vi "AutoReadFile.vi"(8 "error in (no error)":errorcluster, 11 "FileName":string="trajectory.csv") -> (0 "error out":errorcluster, 3 "outTRAJECTORY":T1[](array[typedef]), 4 "Full FIlename":string)   [LabVIEW 2023]
doc: "Create a trajectory from a CSV file. This can be used on a PC or the RoboRIO. Normally the CSV file is created as output from one of the trajectory utility programs. The file could also be created manually or by a custom written program.\n\nParameters:\n - FileName -- Name of the CSV file to read. See file name notes for additional information.\n - Error In -- Input error cluster (optional)\n\nReturns:\n - outTrajectory - Trajectory data structure cluster\n - Error out - returned error cluster\n\nNotes on use:\n -- This routine writes informational messges to the console and to the driver station log.\n\nNotes on file naming:\n -- The file name must include the extention. \".csv\" is not automatically appended to the name. \n -- The file name can be a simple file or an absolute path. If a simple file name is used the default path on the RoboRIO is: \"home:\\lvuser\\natinst\\LabVIEW Data\". On a Windows PC the default path is the LabVIEW default directory. Normally this is: “%HOMEDRIVE%%HOMEPATH%\\Documents\\LabView Data\".\n -- Filenames on the RoboRIO, which runs Linux, are case sensitive.\n\nNotes on file contents:\n -- Blank lines are ignored.\n -- Lines that begin with either #, !, or ' in the first character are considered comments and are ignored. \n -- Other lines are interpretted as comma separated data as follows:\n -- Trajectory time -- seconds\n -- Expected velocity -- meters/sec\n -- Expected acceleration -- meters/sec^2\n -- Expected X position -- meters\n -- Expected Y position -- meters\n -- Expected heading (not necessarily robot orientation) -- radians\n -- Expected curvature (rotational portion of velocity) -- radians/meter\n -- Optional comment string. This ignored when reading file"
uses:
  ClusterTypedef.ctl
  ClusterEnumTypedef.ctl
  <vilib>/Utility/error.llb/whitespace.ctl
  <vilib>/Utility/error.llb/Trim Whitespace One-Sided.vi
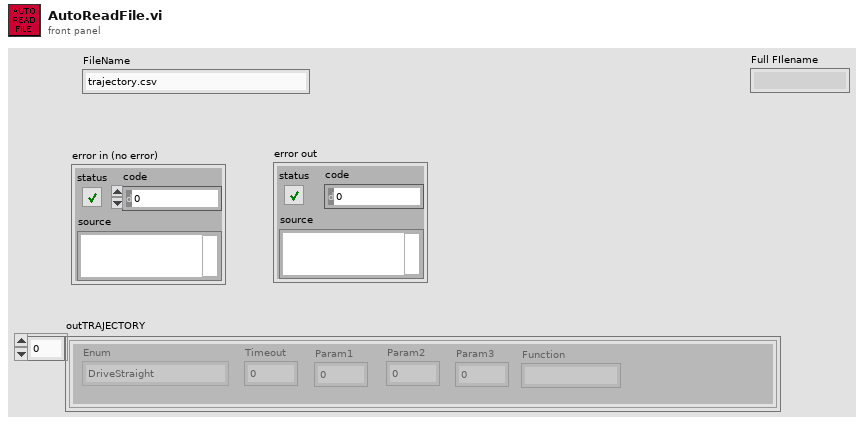
[diagram p1: front panel]
types:
  T1 = typedef "ClusterTypedef.ctl" = cluster{"Enum":T2, "Timeout":dbl, "Param1":dbl, "Param2":dbl, "Param3":dbl, "Function":string}
  T2 = typedef "ClusterEnumTypedef.ctl" = enum16{"DriveStraight", "DriveTurn", "FollowAbsoluteTrajectory", "FollowRelativeTrajectory", "AutoWait", "ElevToRest", "ElevToSource", "ElevToL1", "ElevToL2", "ElevToL3", "ElevToL4", "ElevToAlgae1", "ElevToAlgae2", "ElevCancel", "IntakeCoral", "IntakeAlgae", "IntakeDepositCoral", "IntakeDepositAlgae", "IntakeCancel", "ElevRestWait", "ElevSourceWait", "ElevL1Wait", "ElevL2Wait", "ElevAlgae1Wait", "ElevL3Wait", "ElevAlgae2Wait", "ElevL4Wait"}
  T3 = enum16{"open", "replace", "create", "open or create", "replace or create", "replace or create with confirmation"}
  T4 = typedef "whitespace.ctl" = u16
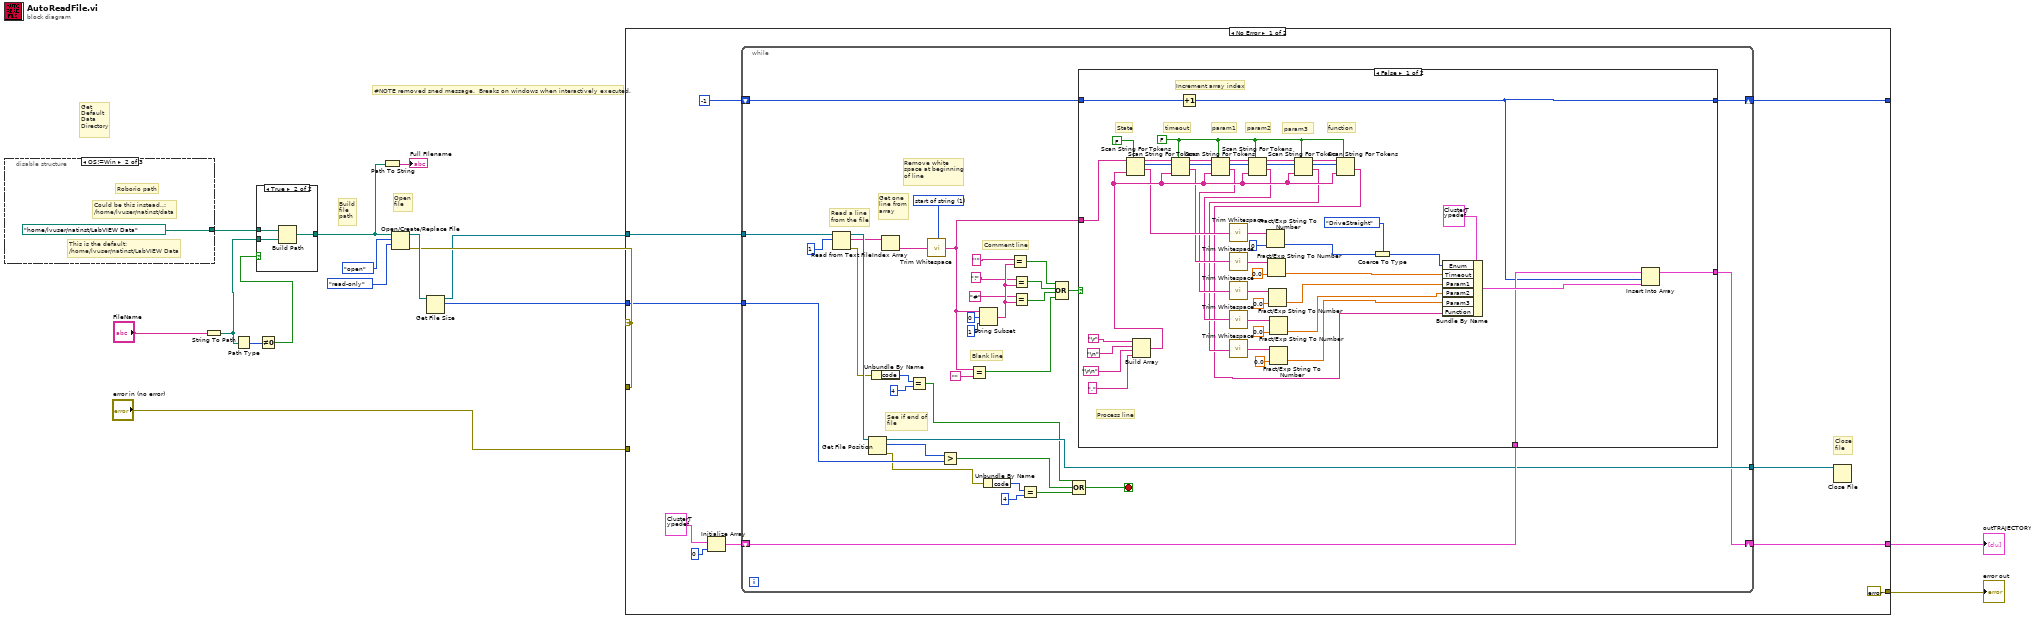
[diagram p0: block diagram]
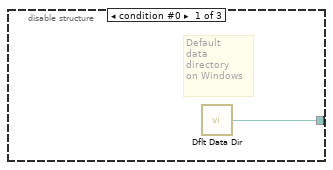
[diagram p3: hidden frame]
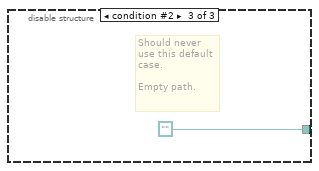
[diagram p4: hidden frame]
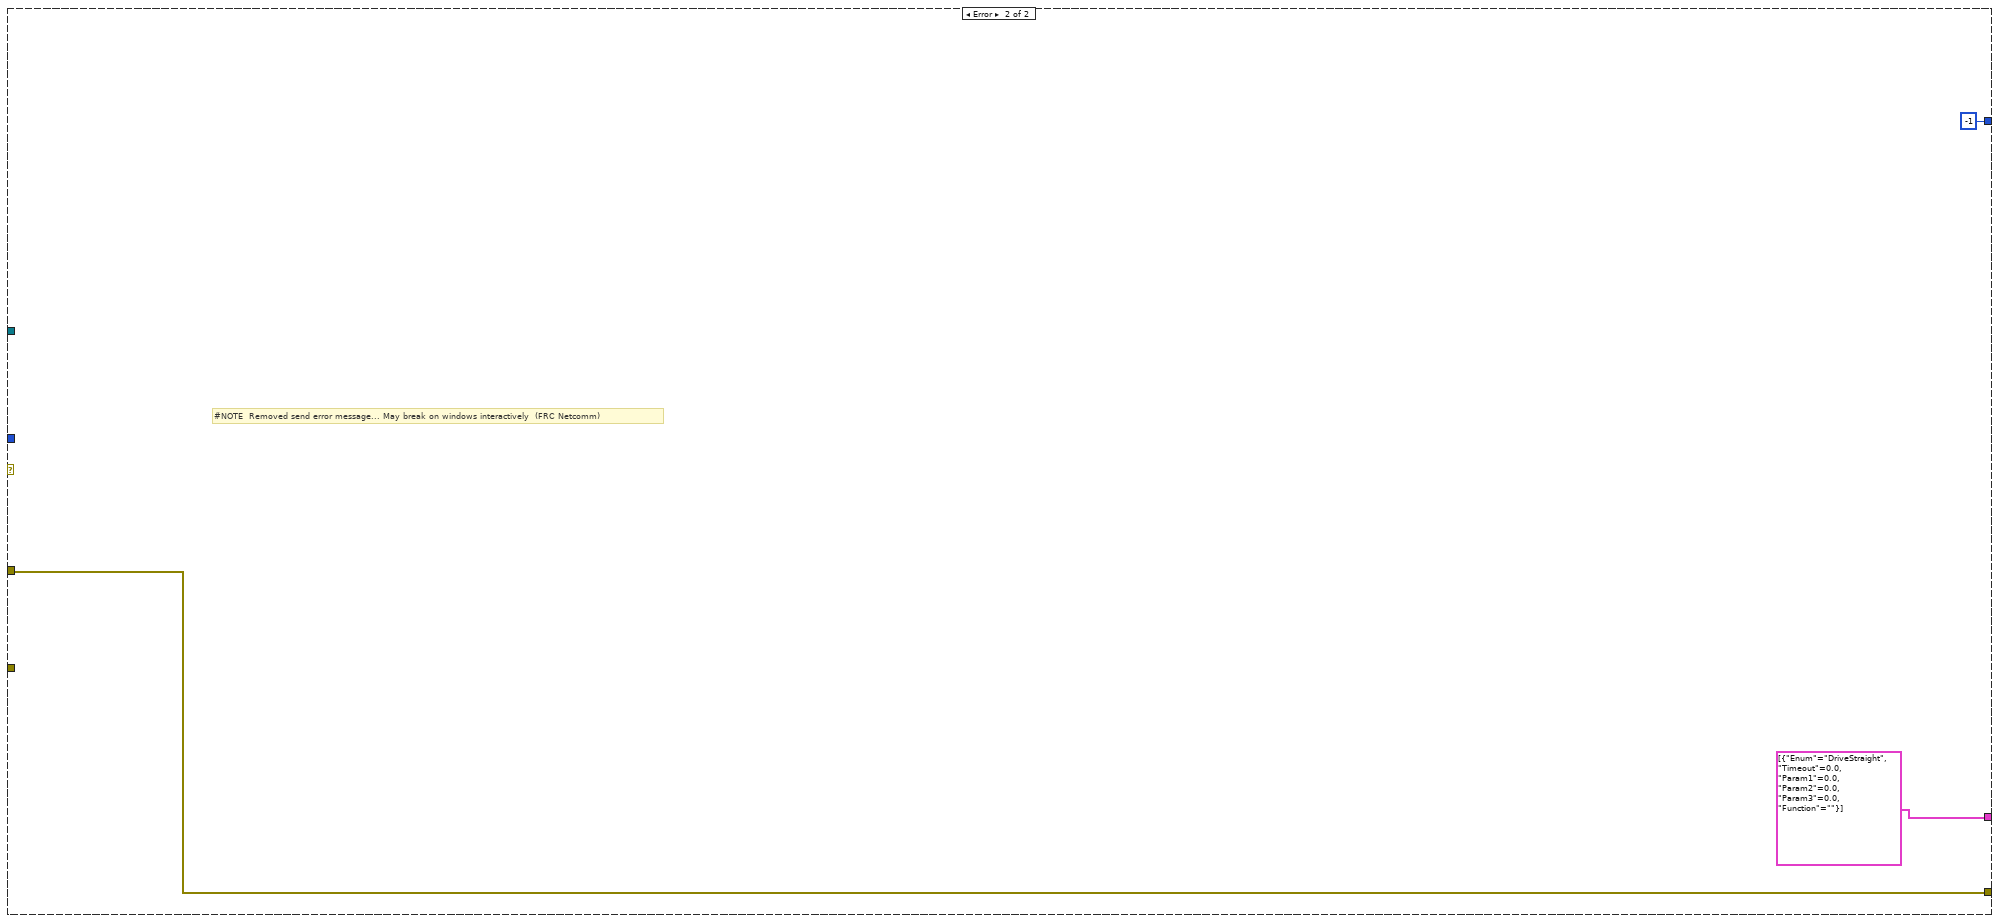
[diagram p6: hidden frame]
diagram:
  # "#NOTE removed sned message.  Breaks on windows when interactively executed."
  # "Get\nDefault\nData\nDirectory"
  # "Open\nfile"
  # "Build\nfile\npath"
  n1 = disable-structure shown="OS!=Win" {
    disable-tunnel: [w17 path "/home/lvuser/natinst/LabVIEW Data" path ""] -> w10
    frame condition #0 {
      # "Default\ndata\ndirectory\non Windows"
      n2 = call <vilib>:"Dflt Data Dir.vi"() -> ("App:Default Data Directory"=w17:path)
    }
    frame condition #1 (active) {
      # "This is the default:\n/home/lvuser/natinst/LabVIEW Data"
      # "Could be this instead..:\n/home/lvuser/natinst/data"
      # "Roborio path"
    }
    frame condition #2 {
      # "Should never\nuse this default\ncase.\n\nEmpty path."
    }
  }
  n3 = String To Path(string="FileName") -> (path=w7:path)
  n4 = Path Type(1:w7) -> (0:w6:i16)
  n5 = Not Equal To 0?(x=w6) -> (x != 0?=w5:bool)
  n6 = case shown="True" w5 {
    tunnel: [w20 w23] -> w13
    tunnel: w10 -> [_ w22]
    tunnel: w7 -> [w20 w21]
    frame False {
    }
    frame True {
      n7 = Build Path(base path=w22, name or relative path=w21) -> (appended path=w23:path)
    }
  }
  n8 = Path To String(path=w13) -> (string=→"Full FIlename":string)
  n9 = Open/Create/Replace File(file path (use dialog)=w13, operation (0:open)=T3."open", access (0:read/write)=enum16{"read/write", "read-only", "write-only"}."read-only") -> (refnum out=w14:refnum<file>, error out=w11:errorcluster)  [unwired: 3 in, 1 out]
  n10 = Get File Size(file=w14) -> (refnum out=w4:refnum<file>, size (in bytes)=w12:i64)  [unwired: 1 in, 1 out]
  n11 = case shown="No Error" w11 {
    tunnel: w4 -> [w33 _]
    tunnel: w12 -> [w31 _]
    tunnel: [w27 i16 -1] -> _
    tunnel: [w26 T1[] [{"Enum"=enum."DriveStraight", "Timeout"=0.0, "Param1"=0.0, "Param2"=0.0, "Param3"=0.0, "Function"=""}] ("Array")] -> w1
    tunnel: w11 -> [_ w120]
    tunnel: [errorcluster {"status"=FALSE, "code"=0, "source"=""} ("error out") w120] -> w9
    tunnel: "error in (no error)" -> [_ _]
    frame No Error {
      # "Close\nfile"
      n12 = Initialize Array(T1 {"Enum"=enum."DriveStraight", "Timeout"=0.0, "Param1"=0.0, "Param2"=0.0, "Param3"=0.0, "Function"=""} ("AutoCluster"), 0 ("dimension size")) -> (w28:T1[])
      n13 = while {
        tunnel: w33 -> [w69]
        tunnel: w31 -> [w65]
        tunnel: [w45] -> w30
        shift-right: [w35] -> w27
        shift-left: i16 -1 -> [w49]
        shift-right: [w34] -> w26
        shift-left: w28 -> [w47]
        stop <- w43 stop-if-true
        w64 = T4 1 items=["both", "start of string", "end of string"] ("location (both)")
        # "Comment line"
        # "Blank line"
        # "Remove white \nspace at beginning\nof line"
        # "Get one\nline from\narray"
        # "Read a line\nfrom the file"
        # "See if end of \nfile"
        n14 = Read from Text File(file (use dialog)=w69, count=1) -> (refnum out=w67:refnum<file>, text=w63:string[], error out=w46:errorcluster)  [unwired: 2 in, 1 out]
        n15 = Get File Position(7:w67) -> (0:w38:errorcluster, 2:w66:i64, 3:w45:refnum<file>)  [unwired: 1 in]
        n16 = Unbundle By Name(w46) -> ("code"=w42:i32)
        n17 = Index Array(array=w63) -> (element=w62:string)  [unwired: 1 in]
        n18 = Equal?(x=w42, y=4) -> (x = y?=w37:bool)
        n19 = call <vilib>:"Trim Whitespace.vi"("string"=w62, "location (both)"=w64) -> ("trimmed string"=w48:string)
        n20 = Greater?(x=w66, y=w65) -> (0:w44:bool)
        n21 = Equal?(x=w48, y="") -> (x = y?=w51:bool)
        n22 = String Subset(string=w48, offset (0)=0, length (rest)=1 ("length (rest)")) -> (substring=w58:string)
        n23 = Unbundle By Name(w38) -> ("code"=w40:i32)
        n24 = Equal?(x="'", y=w58) -> (x = y?=w54:bool)
        n25 = Equal?(x="!", y=w58) -> (x = y?=w53:bool)
        n26 = Equal?(x="#", y=w58) -> (x = y?=w52:bool)
        n27 = Equal?(x=w40, y=4) -> (x = y?=w36:bool)
        n28 = Compound Arithmetic op=OR(w54, w53, w52, w51) -> (w50:bool)
        n29 = Compound Arithmetic op=OR(w37, w44, w36) -> (w43:bool)
        n30 = case shown="False" w50 {
          tunnel: w49 -> [w116 w117]
          tunnel: [w82 w117] -> w35
          tunnel: w48 -> [w81 _]
          tunnel: w47 -> [w84 w118]
          tunnel: [w83 w118] -> w34
          frame False {
            w79 = FALSE ("allow empty tokens? (F)")
            # "function"
            # "param3"
            # "param2"
            # "param1"
            # "timeout"
            # "State"
            # "Increment array index"
            # "Process line"
            n31 = Build Array("\r", "\n", "\r\n", ",") -> (w110:string[])
            n32 = Scan String For Tokens(5:FALSE ("allow empty tokens? (F)"), 6:w110, 9:w81) -> (1:w99:string, 2:w104:i32, 3:w109:string)  [unwired: 3 in, 1 out]
            n33 = Scan String For Tokens(5:w79, 6:w110, 8:w104, 9:w109) -> (1:w98:string, 2:w103:i32, 3:w108:string)  [unwired: 2 in, 1 out]
            n34 = Increment(x=w116) -> (x+1=w82:i16)
            n35 = Scan String For Tokens(5:w79, 6:w110, 8:w103, 9:w108) -> (1:w97:string, 2:w102:i32, 3:w107:string)  [unwired: 2 in, 1 out]
            n36 = call <vilib>:"Trim Whitespace.vi"("string"=w99) -> ("trimmed string"=w78:string)  [unwired: 1 in]
            n37 = call <vilib>:"Trim Whitespace.vi"("string"=w98) -> ("trimmed string"=w93:string)  [unwired: 1 in]
            n38 = call <vilib>:"Trim Whitespace.vi"("string"=w97) -> ("trimmed string"=w89:string)  [unwired: 1 in]
            n39 = Scan String For Tokens(5:w79, 6:w110, 8:w102, 9:w107) -> (1:w96:string, 2:w101:i32, 3:w106:string)  [unwired: 2 in, 1 out]
            n40 = call <vilib>:"Trim Whitespace.vi"("string"=w96) -> ("trimmed string"=w88:string)  [unwired: 1 in]
            n41 = Fract/Exp String To Number(string=w78, default (0 dbl)=0 ("default (0 DBL)")) -> (number=w71:i32)  [unwired: 2 in, 1 out]
            n42 = Fract/Exp String To Number(string=w93, default (0 dbl)=0.0 ("default (0 DBL)")) -> (number=w86:dbl)  [unwired: 2 in, 1 out]
            n43 = Fract/Exp String To Number(string=w89, default (0 dbl)=0.0 ("default (0 DBL)")) -> (number=w80:dbl)  [unwired: 2 in, 1 out]
            n44 = Fract/Exp String To Number(string=w88, default (0 dbl)=0.0 ("default (0 DBL)")) -> (number=w75:dbl)  [unwired: 2 in, 1 out]
            n45 = Scan String For Tokens(5:w79, 6:w110, 8:w101, 9:w106) -> (1:w95:string, 2:w100:i32, 3:w105:string)  [unwired: 2 in, 1 out]
            n46 = call <vilib>:"Trim Whitespace.vi"("string"=w95) -> ("trimmed string"=w87:string)  [unwired: 1 in]
            n47 = Fract/Exp String To Number(string=w87, default (0 dbl)=0.0 ("default (0 DBL)")) -> (number=w74:dbl)  [unwired: 2 in, 1 out]
            n48 = Scan String For Tokens(5:w79, 6:w110, 8:w100, 9:w105) -> (1:w73:string)  [unwired: 2 in, 3 out]
            n49 = Coerce To Type(0:w71, 1:ClusterEnumTypedef."DriveStraight" ("Function")) -> (2:w70:T2)
            n50 = Bundle By Name(cluster=T1 {"Enum"=enum."DriveStraight", "Timeout"=0.0, "Param1"=0.0, "Param2"=0.0, "Param3"=0.0, "Function"=""} ("AutoCluster"), "Enum"=w70, "Timeout"=w86, "Param1"=w80, "Param2"=w75, "Param3"=w74, "Function"=w73) -> (w85:T1)
            n51 = Insert Into Array(array=w84, index=w82, new element=w85) -> (w83:T1[])
          }
          frame True {
            # "Comment -- ignore."
          }
        }
      }
      n52 = Close File(refnum=w30) -> ()  [unwired: 1 in, 2 out]
    }
    frame Error {
      # "#NOTE  Removed send error message... May break on windows interactively  (FRC Netcomm)"
    }
  }
  "error out" <- w9
  "outTRAJECTORY" <- w1
